vi "Data Unpack.vi"(0 "acquisition file to unpack":path, 1 "extraction duration (s)":dbl=2147483647.0, 2 "display?":bool) -> (8 "display":cluster{"y":dbl, dbl, dbl[][]}(graph))   [LabVIEW 2009]
uses:
  <vilib>/Utility/error.llb/DialogType.ctl
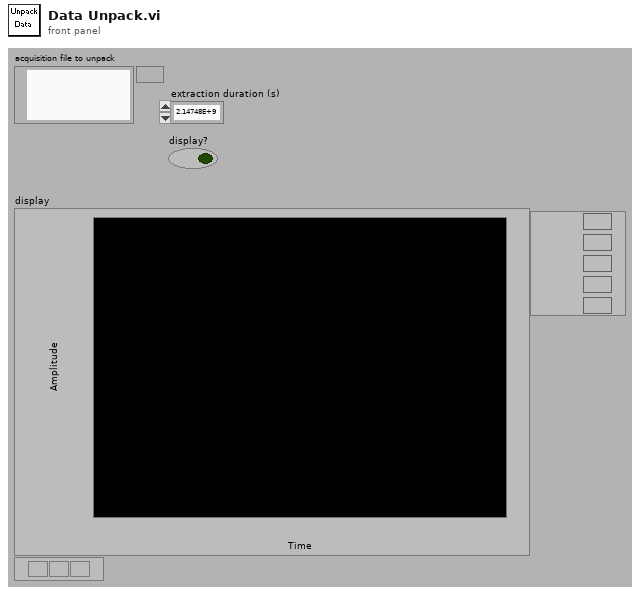
[diagram p1: front panel]
types:
  T1 = typedef "DialogType.ctl" = u16
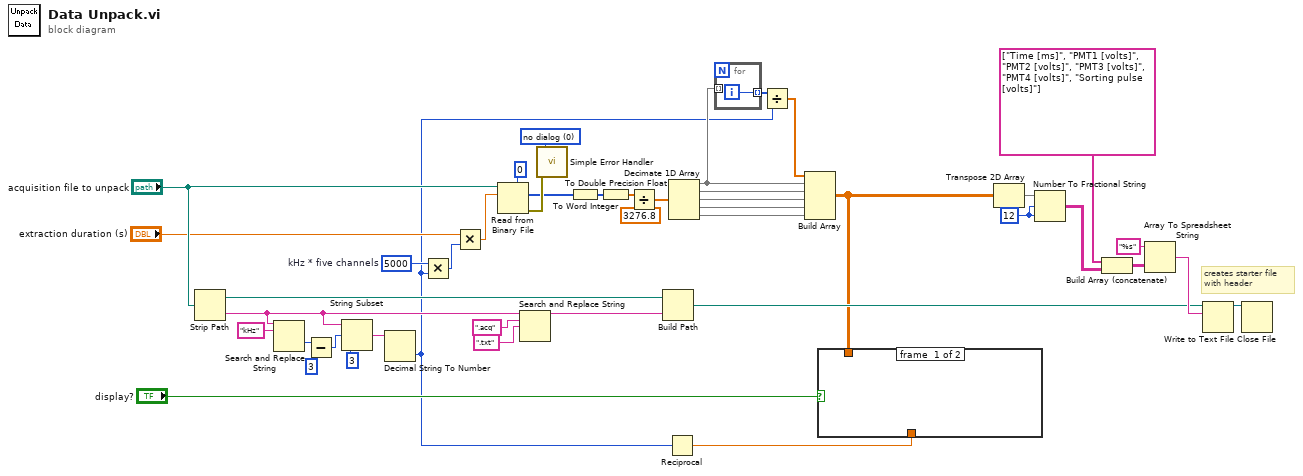
[diagram p0: block diagram]
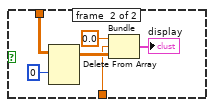
[diagram p2: hidden frame]
diagram:
  w16 = 5000  # kHz * five channels
  w28 = T1 0 items=["no dialog", "OK message", "continue or stop message", "OK message + warnings", "continue/stop + warnings"] ("type of dialog (OK msg:1)")
  w39 = i16 12 ("precision (6)")
  # "creates starter file\nwith header"
  n1 = Strip Path(path="acquisition file to unpack") -> (stripped path=w23:path, name=w20:string)
  n2 = Search and Replace String(input string=w20, search string="kHz") -> (offset past replacement=w30:i32)  [unwired: 6 in, 3 out]
  n3 = Subtract(x=w30, y=3 ("length (rest)")) -> (x-y=w26:i32)
  n4 = String Subset(string=w20, offset (0)=w26, length (rest)=3 ("length (rest)")) -> (substring=w25:string)
  n5 = Decimal String To Number(string=w25) -> (number=w2:i32)  [unwired: 2 in, 1 out]
  n6 = Multiply(x=w16, y=w2) -> (x*y=w15:i32)
  n7 = Multiply(x="extraction duration (s)", y=w15) -> (x*y=w14:dbl)
  n8 = Read from Binary File(5:u32 0 ("count"), 10:w14, 11:"acquisition file to unpack") -> (0:w27:errorcluster, 2:w6:u32[])  [unwired: 3 in, 2 out]
  n9 = Search and Replace String(input string=w20, search string=".acq", replace string=".txt" ("replace string (\"\")")) -> (result string=w19:string)  [unwired: 5 in, 3 out]
  n10 = call <vilib>:"Simple Error Handler.vi"("type of dialog (OK msg:1)"=w28, "error in (no error)"=w27) -> ()  [unwired: 3 in, 5 out]
  n11 = To Word Integer(number=w6) -> (16bit integer=w8:i16[])
  n12 = To Double Precision Float(number=w8) -> (double precision float=w9:dbl[])
  n13 = Divide(x=w9, y=3276.8) -> (x/y=w5:dbl[])
  n14 = Build Path(base path=w23, name or relative path=w19) -> (appended path=w18:path)
  n15 = Reciprocal(x=w2) -> (1/x=w1:dbl)
  n16 = Decimate 1D Array(w5) -> (w12:dbl[], w40:dbl[], w41:dbl[], w42:dbl[], w43:dbl[])
  n17 = for {
    tunnel: w12 -> [_] mode=indexing
    tunnel: [w45] -> w11 mode=indexing
    i -> [w45]
  }
  n18 = Divide(x=w11, y=w2) -> (x/y=w4:dbl[])
  n19 = Build Array(w4, w12, w40, w41, w42, w43) -> (w3:dbl[][])
  n20 = case shown="True" "display?" {
    tunnel: w3 -> [_ w51]
    tunnel: w1 -> [_ w48]
    frame #0 {
    }
    frame #1 {
      n21 = Delete From Array(array=w51, index (row)=0) -> (array with subset deleted=w49:dbl[][])  [unwired: 2 in, 1 out]
      n22 = Bundle("y"=0.0, w48, w49) -> (→"display":cluster{"y":dbl, dbl, dbl[][]})  [unwired: 1 in]
    }
  }
  n23 = Transpose 2D Array(2D array=w3) -> (transposed array=w24:dbl[][])
  n24 = Number To Fractional String(number=w24, width (-)=w39, precision (6)=w39) -> (F-format string=w38:string[][])  [unwired: 1 in]
  n25 = Build Array (concatenate)(string[] ["Time [ms]", "PMT1 [volts]", "PMT2 [volts]", "PMT3 [volts]", "PMT4 [volts]", "Sorting pulse [volts]"] ("column titles"), w38) -> (w17:string[][])
  n26 = Array To Spreadsheet String(array=w17, 3:"%s" ("format string")) -> (spreadsheet string=w35:string)  [unwired: 1 in]
  n27 = Write to Text File(file (use dialog)=w18, text=w35) -> (refnum out=w37:refnum<file>)  [unwired: 2 in, 2 out]
  n28 = Close File(refnum=w37) -> ()  [unwired: 1 in, 2 out]
